vi "testschleife.vi"() -> ()   [LabVIEW 2010]
panel:
  out "Array (Ausgang)":i32[](array[numeric])
  out "Angehängtes Array":i32[][](array[numeric])
  in  "Array 4":bool[][](array[boolean])=[[FALSE, FALSE], [FALSE, FALSE], [FALSE, FALSE], [FALSE, FALSE]]
  out "Array 2":dbl[][](array[numeric])
  out "Zyklusnummern":dbl[](array[numeric])
  out "Zykluszeiten":dbl[](array[numeric])
  out "Elapsed Time (s)":dbl caption="Verstrichene Zeit (s)"
  in  "Stopp 2":bool
  out "x*y":i16[](array[numeric])
  out "Erstes Teil-Array":bool[](array[boolean])
  out "Zweites Teil-Array":bool[](array[boolean])
  in  "DIO1 \"aus\"":bool
  out "Array":bool[](array[boolean])
  out "Present (s)":dbl caption="Aktuell (s)"
  in  "Stopp":bool
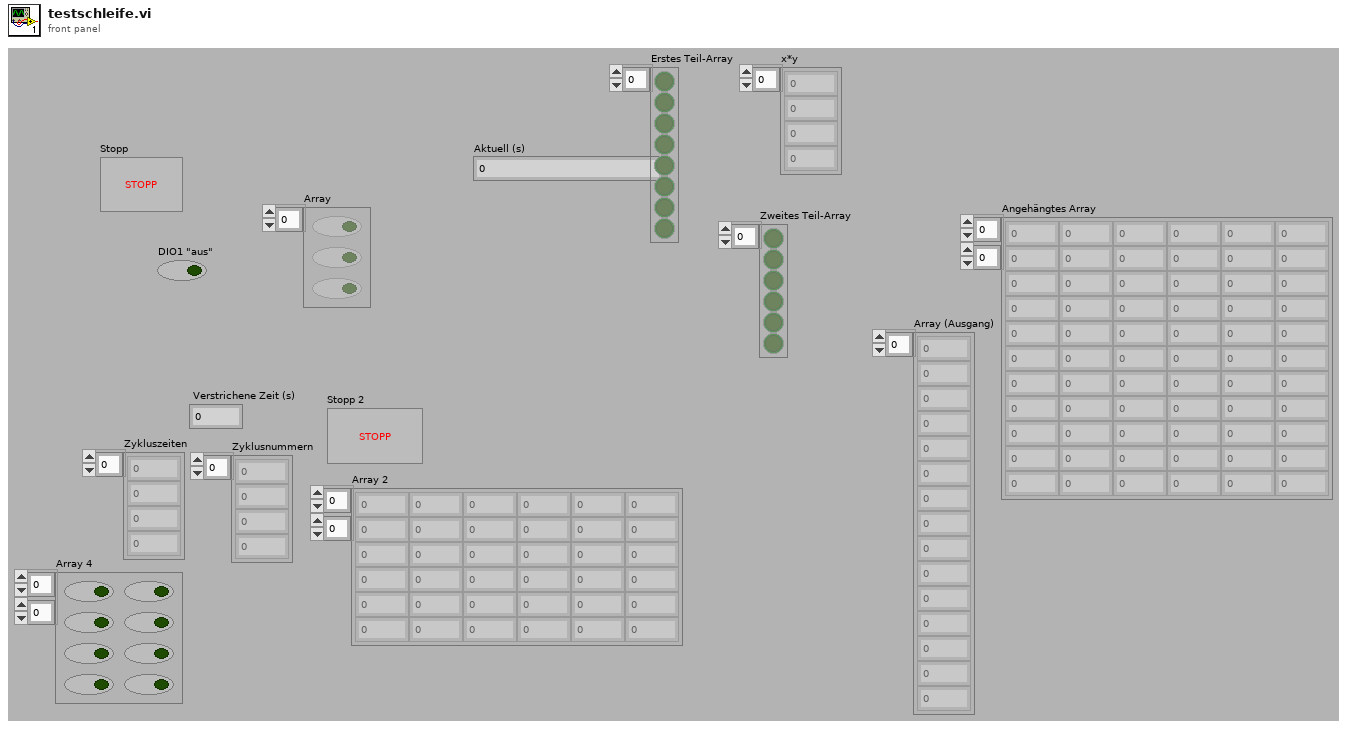
[diagram p1: front panel]
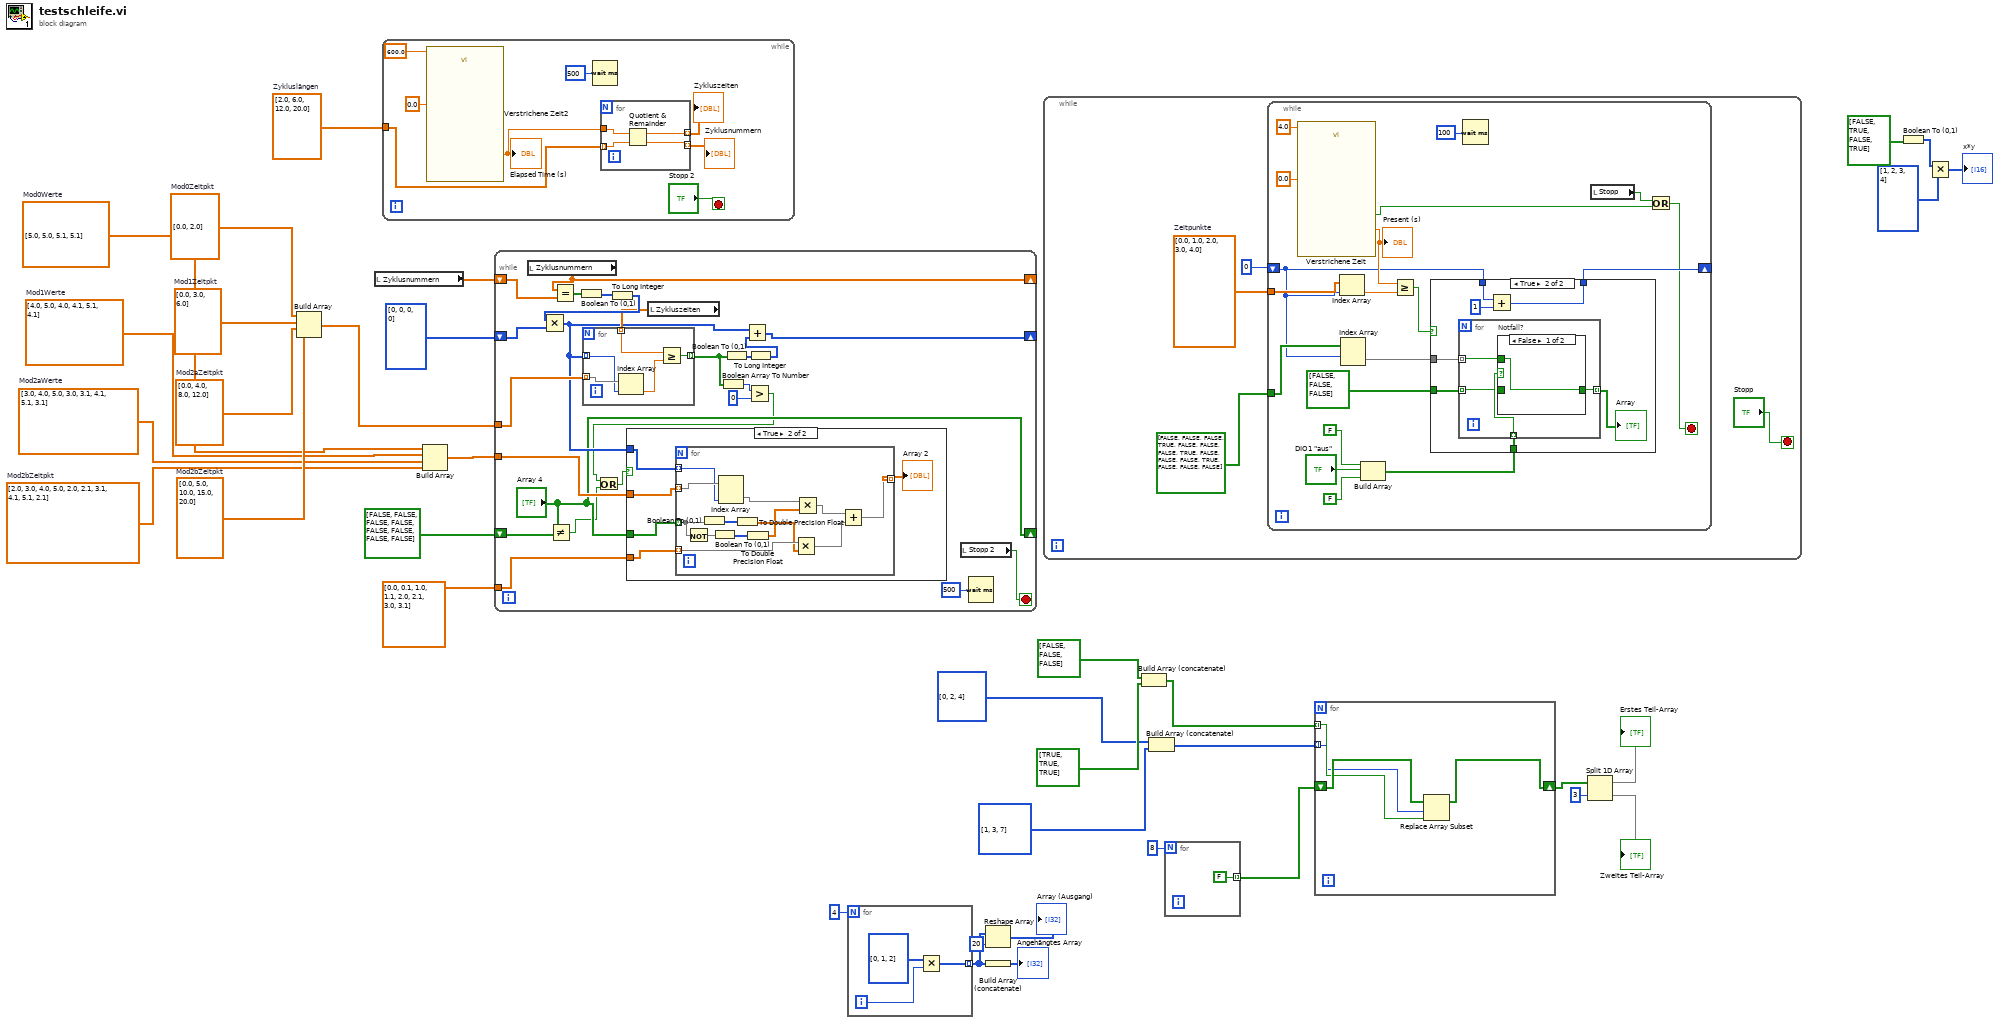
[diagram p0: block diagram]
diagram:
  w11 = dbl[][] [[2.0, 3.0, 4.0, 5.0, 2.0], [2.1, 3.1, 4.1, 5.1, 2.1]]  # Mod2bZeitpkt
  w12 = dbl[][] [[3.0, 4.0, 5.0, 3.0], [3.1, 4.1, 5.1, 3.1]]  # Mod2aWerte
  w13 = dbl[][] [[4.0, 5.0, 4.0], [4.1, 5.1, 4.1]]  # Mod1Werte
  w14 = dbl[][] [[5.0, 5.0], [5.1, 5.1]]  # Mod0Werte
  w15 = dbl[] [2.0, 6.0, 12.0, 20.0]  # Zykluslängen
  w17 = dbl[] [0.0, 5.0, 10.0, 15.0, 20.0]  # Mod2bZeitpkt
  w18 = dbl[] [0.0, 4.0, 8.0, 12.0]  # Mod2aZeitpkt
  w19 = dbl[] [0.0, 3.0, 6.0]  # Mod1Zeitpkt
  w20 = dbl[] [0.0, 2.0]  # Mod0Zeitpkt
  n1 = Build Array(w20, w19, w18, w17) -> (w16:dbl[][])
  n2 = local read "Zyklusnummern"() -> (w8:dbl[])
  n3 = while {
    tunnel: w15 -> [w39]
    stop <- "Stopp 2" stop-if-true
    n4 = call "Verstrichene Zeit2"("Time Target (s)"=600.0, "Set Start Time (s)"=0.0) -> ("Elapsed Time (s)"=w40:dbl)  [unwired: 10 in, 7 out]
    "Elapsed Time (s)" <- w40
    n5 = Wait (ms)(milliseconds to wait=u32 500 ("Zu wartende ms")) -> ()  [unwired: 1 out]
    n6 = for {
      tunnel: w40 -> [w48]
      tunnel: w39 -> [w47] mode=indexing
      tunnel: [w46] -> w38 mode=indexing
      tunnel: [w45] -> w37 mode=indexing
      n7 = Quotient & Remainder(x=w48, y=w47) -> (x-y*floor(x/y)=w46:dbl, floor(x/y)=w45:dbl)
    }
    "Zykluszeiten" <- w38
    "Zyklusnummern" <- w37
  }
  n8 = Build Array(w14, w13, w12, w11) -> (w10:dbl[][][])
  n9 = while {
    tunnel: w16 -> [w64]
    tunnel: w10 -> [w56]
    shift-right: [w60] -> _
    shift-left: i32[] [0, 0, 0, 0] -> [w66]
    shift-right: [w69] -> _
    shift-left: w8 -> [w70]
    tunnel: dbl[][] [[0.0, 0.1], [1.0, 1.1], [2.0, 2.1], [3.0, 3.1]] -> [w54]
    shift-right: ["Array 4"] -> _
    shift-left: bool[][] [[FALSE, FALSE], [FALSE, FALSE], [FALSE, FALSE], [FALSE, FALSE]] ("Array 4") -> [w52]
    stop <- w71 stop-if-true
    n10 = local read "Zyklusnummern"() -> (w69:dbl[])
    n11 = Not Equal?(x="Array 4", y=w52) -> (x != y?=w50:bool)
    n12 = Equal?(x=w69, y=w70) -> (x = y?=w68:bool[])
    n13 = Boolean To (0,1)(Boolean=w68) -> (0, 1=w67:i16[])
    n14 = To Long Integer(number=w67) -> (32bit integer=w65:i32[])
    n15 = Multiply(x=w65, y=w66) -> (x*y=w55:i32[])
    n16 = local read "Zykluszeiten"() -> (w63:dbl[])
    n17 = for {
      tunnel: w55 -> [w94] mode=indexing
      tunnel: w64 -> [w95] mode=indexing
      tunnel: w63 -> [w93] mode=indexing
      tunnel: [w91] -> w59 mode=indexing
      n18 = Index Array(array=w95, index=w94) -> (element=w92:dbl)
      n19 = Greater Or Equal?(x=w93, y=w92) -> (x >= y?=w91:bool)
    }
    n20 = Boolean Array To Number(Boolean array=w59) -> (number=w58:u32)
    n21 = Boolean To (0,1)(Boolean=w59) -> (0, 1=w62:i16[])
    n22 = Greater?(x=w58, y=u32 0) -> (0:w51:bool)
    n23 = Or(x=w51, y=w50) -> (x .or. y?=w49:bool)
    n24 = case shown="True" w49 {
      tunnel: w56 -> [_ w77]
      tunnel: w55 -> [_ w76]
      tunnel: "Array 4" -> [_ w73]
      tunnel: w54 -> [_ w74]
      frame False {
      }
      frame True {
        n25 = for {
          tunnel: w77 -> [w90] mode=indexing
          tunnel: w76 -> [w89] mode=indexing
          tunnel: [w82] -> w75 mode=indexing
          tunnel: w74 -> [w80] mode=indexing
          tunnel: w73 -> [w87] mode=indexing
          n26 = Not(x=w87) -> (.not. x?=w85:bool[])
          n27 = Boolean To (0,1)(Boolean=w87) -> (0, 1=w88:i16[])
          n28 = Boolean To (0,1)(Boolean=w85) -> (0, 1=w86:i16[])
          n29 = Index Array(array=w90, index (col)=w89) -> (element=w81:dbl[])  [unwired: 1 in]
          n30 = To Double Precision Float(number=w88) -> (double precision float=w79:dbl[])
          n31 = To Double Precision Float(number=w86) -> (double precision float=w78:dbl[])
          n32 = Multiply(x=w80, y=w79) -> (x*y=w83:dbl[])
          n33 = Multiply(x=w81, y=w78) -> (x*y=w84:dbl[])
          n34 = Add(x=w84, y=w83) -> (x+y=w82:dbl[])
        }
        "Array 2" <- w75
      }
    }
    n35 = To Long Integer(number=w62) -> (32bit integer=w61:i32[])
    n36 = Add(x=w55, y=w61) -> (x+y=w60:i32[])
    n37 = local read "Stopp 2"() -> (w71:bool)
    n38 = Wait (ms)(milliseconds to wait=u32 500 ("Zu wartende ms")) -> ()  [unwired: 1 out]
  }
  n39 = for {
    N: 4 -> [_]
    tunnel: [w96] -> w3 mode=indexing
    i -> [w97]
    n40 = Multiply(x=i32[] [0, 1, 2], y=w97) -> (x*y=w96:i32[])
  }
  n41 = Reshape Array(w3, 20 ("Dimension")) -> (→"Array (Ausgang)":i32[])
  n42 = Build Array (concatenate)(w3) -> (→"Angehängtes Array":i32[][])
  n43 = while {
    stop <- "Stopp" stop-if-true
    w100 = dbl[] [0.0, 1.0, 2.0, 3.0, 4.0]  # Zeitpunkte
    n44 = while {
      tunnel: w100 -> [w118]
      tunnel: bool[][] [[FALSE, FALSE, FALSE], [TRUE, FALSE, FALSE], [FALSE, TRUE, FALSE], [FALSE, FALSE, TRUE], [FALSE, FALSE, FALSE]] -> [w117]
      shift-right: [w112] -> _
      shift-left: 0 -> [w113]
      stop <- w103 stop-if-true
      n45 = call "Verstrichene Zeit"("Time Target (s)"=4.0, "Set Start Time (s)"=0.0) -> ("Elapsed Time (s)"=w116:dbl, "Time has Elapsed"=w104:bool)  [unwired: 10 in, 6 out]
      "Present (s)" <- w116
      n46 = Index Array(array=w118, index=w113) -> (element=w115:dbl)
      n47 = Index Array(array=w117, index (row)=w113) -> (element=w111:bool[])  [unwired: 1 in]
      n48 = Build Array(FALSE, "DIO1 \"aus\"", FALSE) -> (w107:bool[])
      n49 = Greater Or Equal?(x=w116, y=w115) -> (x >= y?=w114:bool)
      n50 = case shown="True" w114 {
        tunnel: w113 -> [w122 w129]
        tunnel: [w122 w127] -> w112
        tunnel: w111 -> [_ w124]
        tunnel: w107 -> [_ w125]
        tunnel: bool[] [FALSE, FALSE, FALSE] -> [_ w126]
        frame False {
        }
        frame True {
          n51 = for {
            tunnel: w126 -> [w131] mode=indexing
            tunnel: w125 -> [w133] mode=indexing
            tunnel: w124 -> [w132] mode=indexing
            tunnel: [w130] -> w123 mode=indexing
            n52 = case "Notfall?" shown="False" w133 {
              tunnel: w132 -> [w134 _]
              tunnel: w131 -> [_ w135]
              tunnel: [w134 w135] -> w130
              frame False {
              }
              frame True {
              }
            }
          }
          "Array" <- w123
          n53 = Add(x=w129, y=1) -> (x+y=w127:i32)
        }
      }
      n54 = Wait (ms)(milliseconds to wait=u32 100 ("Zu wartende ms")) -> ()  [unwired: 1 out]
      n55 = local read "Stopp"() -> (w105:bool)
      n56 = Or(x=w105, y=w104) -> (x .or. y?=w103:bool)
    }
  }
  n57 = Build Array (concatenate)(bool[] [FALSE, FALSE, FALSE], bool[] [TRUE, TRUE, TRUE]) -> (w32:bool[])
  n58 = Build Array (concatenate)(i32[] [0, 2, 4], i32[] [1, 3, 7]) -> (w31:i32[])
  n59 = for {
    N: 8 -> [_]
    tunnel: [FALSE] -> w26 mode=indexing
  }
  n60 = for {
    tunnel: w32 -> [w139] mode=indexing
    tunnel: w31 -> [w138] mode=indexing
    shift-right: [w137] -> w30
    shift-left: w26 -> [w140]
    n61 = Replace Array Subset(array=w140, new element=w139, index=w138) -> (w137:bool[])
  }
  n62 = Split 1D Array(array=w30, index=3 ("Index")) -> (first subarray=→"Erstes Teil-Array":bool[], second subarray=→"Zweites Teil-Array":bool[])
  n63 = Boolean To (0,1)(Boolean=bool[] [FALSE, TRUE, FALSE, TRUE]) -> (0, 1=w23:i16[])
  n64 = Multiply(x=w23, y=i16[] [1, 2, 3, 4]) -> (x*y=→"x*y":i16[])
